vi "StudentScope - Voltage Scaling.vi"(0 "CH A Vert Pos":sgl caption="Position", 1 "CH B Vert Pos":sgl caption="Position", 2 "CH A Zero Pos":bool, 3 "CH B Zero Pos":bool, 4 "CH A Scale":u32, 5 "CH B Scale":u32, 7 "CH A Center":bool, 8 "Knob A Refnum":refnum<vi>, 9 "CH B Center":bool, 10 "Knob B Refnum":refnum<vi>, 12 "Raw Y Values":dbl[][](array[numeric])) -> (16 "Scaled Y Values":dbl[][](array[numeric]))   [LabVIEW 2015]
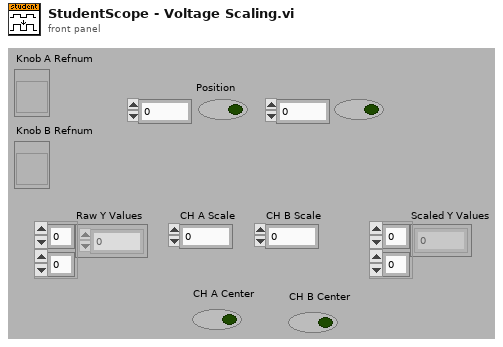
[diagram p1: front panel]
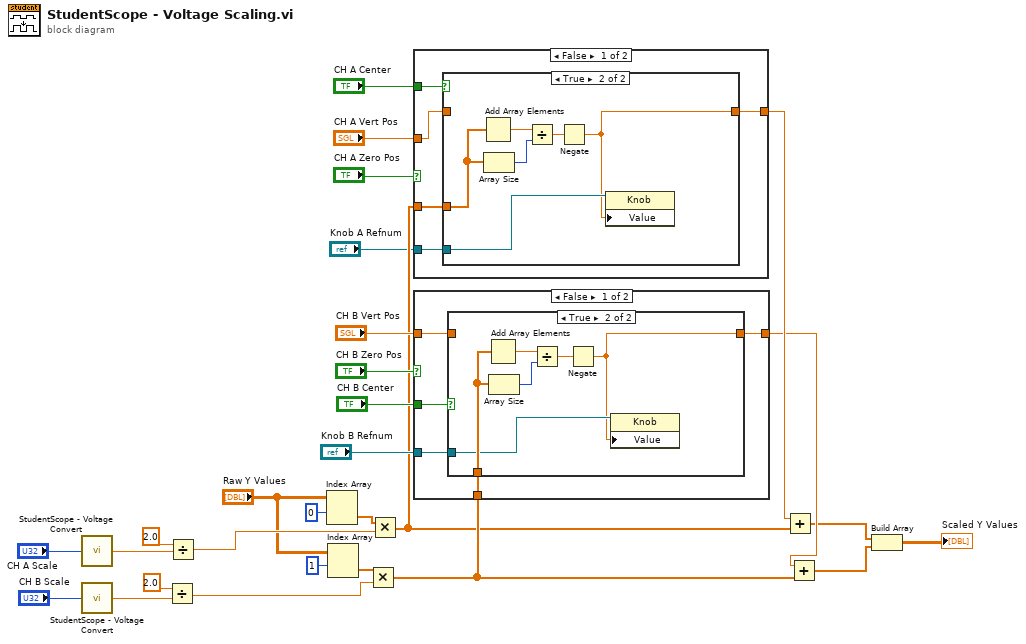
[diagram p0: block diagram]
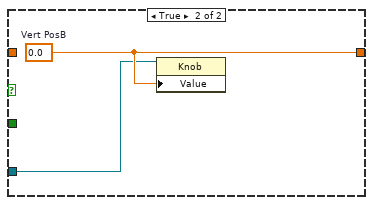
[diagram p3: hidden frame]
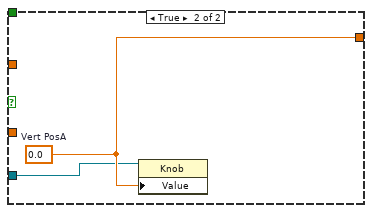
[diagram p5: hidden frame]
diagram:
  n1 = call "StudentScope - Voltage Convert.vi"("CH A Scale"="CH A Scale") -> ("Scaled Voltage"=w20:dbl)
  n2 = call "StudentScope - Voltage Convert.vi"("CH A Scale"="CH B Scale") -> ("Scaled Voltage"=w19:dbl)
  n3 = Divide(x=2.0, y=w19) -> (x/y=w27:dbl)
  n4 = Divide(x=2.0, y=w20) -> (x/y=w14:dbl)
  n5 = Index Array(array="Raw Y Values", index (row)=0 ("index")) -> (element=w15:dbl[])  [unwired: 1 in]
  n6 = Index Array(array="Raw Y Values", index (row)=1 ("index")) -> (element=w12:dbl[])  [unwired: 1 in]
  n7 = Multiply(x=w12, y=w27) -> (x*y=w4:dbl[])
  n8 = Multiply(x=w15, y=w14) -> (x*y=w2:dbl[])
  n9 = case shown="False" "CH A Zero Pos" {
    tunnel: "CH A Vert Pos" -> [w29 _]
    tunnel: [w30 w42] -> w10
    tunnel: "CH A Center" -> [w31 _]
    tunnel: w2 -> [w32 _]
    tunnel: "Knob A Refnum" -> [w33 w41]
    frame False {
      n10 = case shown="True" w31 {
        tunnel: w33 -> [_ w38]
        tunnel: [w34 w35] -> w30
        tunnel: w32 -> [_ w37]
        tunnel: w29 -> [w34 _]
        frame False {
        }
        frame True {
          n11 = Add Array Elements(numeric array=w37) -> (sum=w40:dbl)
          n12 = Array Size(array=w37) -> (size(s)=w39:i32)
          n13 = Divide(x=w40, y=w39) -> (x/y=w36:dbl)
          n14 = Negate(x=w36) -> (-x=w35:dbl)
          n15 = property class="Knob"(reference=w38, "Value"=w35) -> ()  [unwired: 1 in, 2 out]
        }
      }
    }
    frame True {
      w42 = sgl 0.0  # Vert PosA
      n16 = property class="Knob"(reference=w41, "Value"=w42) -> ()  [unwired: 1 in, 2 out]
    }
  }
  n17 = case shown="False" "CH B Zero Pos" {
    tunnel: "CH B Vert Pos" -> [w47 _]
    tunnel: [w43 w56] -> w9
    tunnel: "CH B Center" -> [w45 _]
    tunnel: w4 -> [w46 _]
    tunnel: "Knob B Refnum" -> [w44 w55]
    frame False {
      n18 = case shown="True" w45 {
        tunnel: w47 -> [w48 _]
        tunnel: w46 -> [_ w52]
        tunnel: w44 -> [_ w51]
        tunnel: [w48 w49] -> w43
        frame False {
        }
        frame True {
          n19 = Add Array Elements(numeric array=w52) -> (sum=w54:dbl)
          n20 = Array Size(array=w52) -> (size(s)=w53:i32)
          n21 = Divide(x=w54, y=w53) -> (x/y=w50:dbl)
          n22 = Negate(x=w50) -> (-x=w49:dbl)
          n23 = property class="Knob"(reference=w51, "Value"=w49) -> ()  [unwired: 1 in, 2 out]
        }
      }
    }
    frame True {
      w56 = sgl 0.0  # Vert PosB
      n24 = property class="Knob"(reference=w55, "Value"=w56) -> ()  [unwired: 1 in, 2 out]
    }
  }
  n25 = Add(x=w10, y=w2) -> (x+y=w7:dbl[])
  n26 = Add(x=w9, y=w4) -> (x+y=w8:dbl[])
  n27 = Build Array(w7, w8) -> (→"Scaled Y Values":dbl[][])
